vi "Write number_of_tactics.vi"(8 "error in (no error)":errorcluster, 10 "number_of_tactics":i32=3, 11 "BallPlacementPasserRole in":refnum<class "BallPlacementPasserRole.lvclass">) -> (0 "error out":errorcluster, 3 "BallPlacementPasserRole out":refnum<class "BallPlacementPasserRole.lvclass">)   [LabVIEW 2021, in "BallPlacementPasserRole.lvclass"]
uses:
  BallPlacementPasserRole.lvclass
  BallPlacementPasserRole.lvclass/BallPlacementPasserRole.ctl
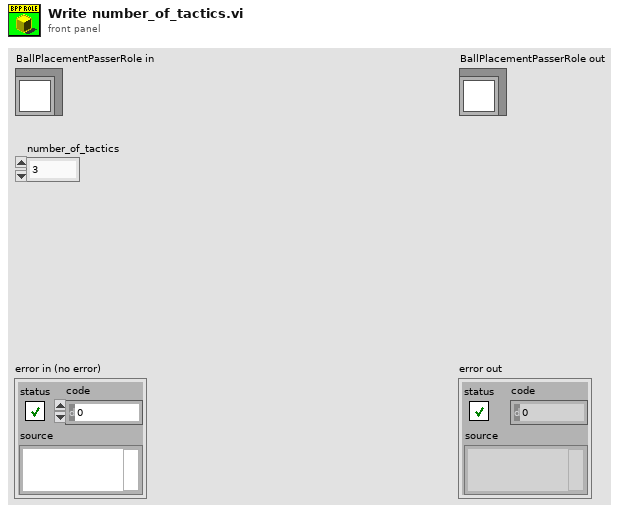
[diagram p1: front panel]
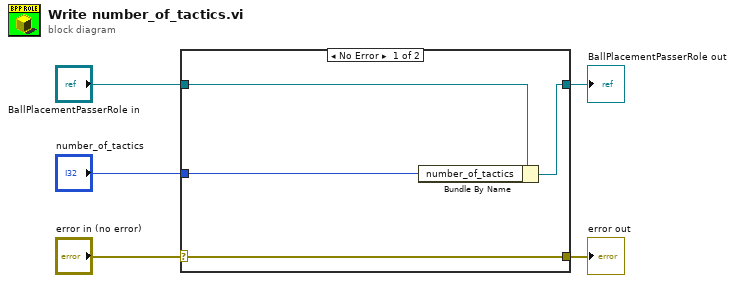
[diagram p0: block diagram]
diagram:
  n1 = case shown="No Error" "error in (no error)" {
    selector: "error in (no error)" -> [w9 w10]
    tunnel: [w9 w10] -> w4
    tunnel: [w7 w11] -> w2
    tunnel: "BallPlacementPasserRole in" -> [w8 w11]
    tunnel: "number_of_tactics" -> [w6 _]
    frame No Error {
      n2 = Bundle By Name(cluster=w8, "number_of_tactics"=w6) -> (w7:refnum<class "BallPlacementPasserRole.lvclass">)
    }
    frame Error {
    }
  }
  "error out" <- w4
  "BallPlacementPasserRole out" <- w2
